vi "Register Elements.vi"(8 "error in (no error)":errorcluster, 11 "PluginGUI in":refnum<class "PluginGUI.lvclass">) -> (0 "error out":errorcluster, 3 "PluginGUI out":refnum<class "PluginGUI.lvclass">)   [LabVIEW 2020, in "VolatusGUI.lvlib" / "PluginGUI.lvclass"]
uses:
  PluginGUI.lvclass
  C:/dev/lv20CE/relink/lv-volatus/Volatus/Module/Module.lvclass
  Volatus/Module/Module.lvclass/Module.ctl
  PluginGUI.lvclass/PluginGUI.ctl
  Volatus/Module/Module.lvclass
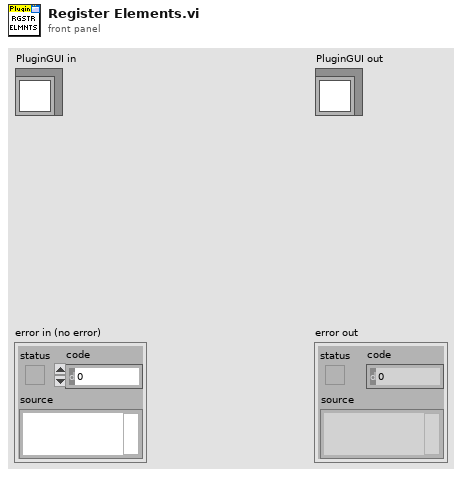
[diagram p1: front panel]
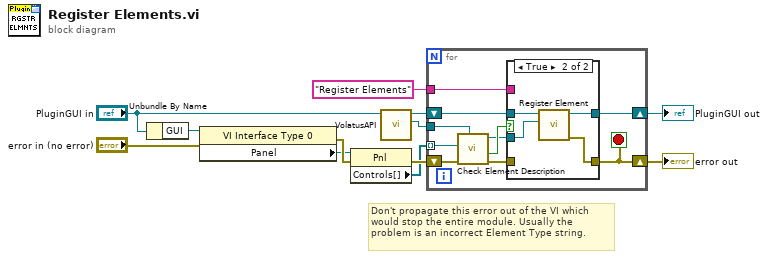
[diagram p0: block diagram]
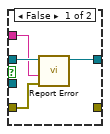
[diagram p2: hidden frame]
diagram:
  # "Don't propagate this error out of the VI which would stop the entire module. Usually the problem is an incorrect Element Type string."
  n1 = Unbundle By Name("PluginGUI in") -> ("GUI"=w11:refnum<vi>)
  n2 = property class="VI Interface Type 0"(reference=w11, error in="error in (no error)") -> (error out=w12:errorcluster, "Panel"=w10:refnum<vi>)  [unwired: 1 out]
  n3 = property class="Pnl"(reference=w10, error in=w12) -> (error out=w9:errorcluster, "Controls[]"=w8:refnum<vi>[])  [unwired: 1 out]
  n4 = call "VolatusAPI.vi"("Module in"="PluginGUI in") -> ("VolatusAPI"=w6:refnum<class "VolatusAPI.lvclass">, "Module out"=w7:refnum<class "PluginGUI.lvclass">)  [unwired: 9 in]
  n5 = for {
    shift-right: [w19] -> w3
    shift-left: w9 -> [w22]
    tunnel: w8 -> [w15] mode=indexing
    shift-right: [w20] -> w4
    shift-left: w7 -> [w21]
    tunnel: w6 -> [w18]
    tunnel: "Register Elements" -> [w13]
    stop <- w19 stop-if-true
    n6 = call "Check Element Description.vi"("VolatusAPI"=w18, "error in (no error)"=w22, "Ref"=w15) -> ("error out"=w16:errorcluster, "Register"=w17:bool, "Element"=w14:refnum<class "GUI Element.lvclass">)  [unwired: 6 in]
    n7 = case shown="True" w17 {
      tunnel: w14 -> [_ w28]
      tunnel: w21 -> [w26 w30]
      tunnel: w16 -> [w24 _]
      tunnel: [_ w27] -> w19
      tunnel: [w25 w29] -> w20
      tunnel: w13 -> [w23 _]
      frame False {
        n8 = call "Report Error.vi"("error in (no error)"=w24, "Message (None)"=w23, "Module in"=w26) -> ("Module out"=w25:refnum<class "PluginGUI.lvclass">)  [unwired: 7 in, 1 out]
      }
      frame True {
        n9 = call "Register Element.vi"("GUI Element"=w28, "PluginGUI in"=w30) -> ("error out"=w27:errorcluster, "PluginGUI out"=w29:refnum<class "PluginGUI.lvclass">)  [unwired: 8 in]
      }
    }
  }
  "error out" <- w3
  "PluginGUI out" <- w4
